vi "Material-ConfigPage-Launch.vi"(0 "Configuration Page VI Filepath":path, 5 "Config Dialog Messenger":refnum<class "FTW-Messenger-Actor.lvclass">, 11 "error in":errorcluster) -> (4 "PageID":string, 6 "Initialized?":bool, 8 "Page Messenger":refnum<class "FTW-Messenger-Actor.lvclass">, 15 "error out":errorcluster)   [LabVIEW 2013, in "Material-ConfigPage.lvclass"]
uses:
  Material-ConfigPage.lvclass
  Reuse Library/featherweight/Core/Messaging/Messenger.Actor/FTW-Messenger-Actor.lvclass
  Material-ConfigPage.lvclass/Material-ConfigPage.ctl
  Reuse Library/featherweight/Core/Messaging/Messenger/FTW-Messenger.lvclass
panel:
  # "Inputs"
  # "Outputs"
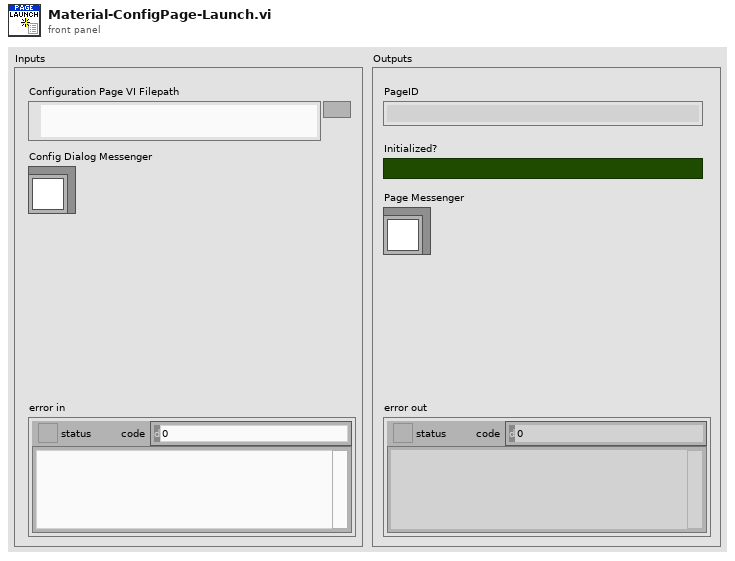
[diagram p1: front panel]
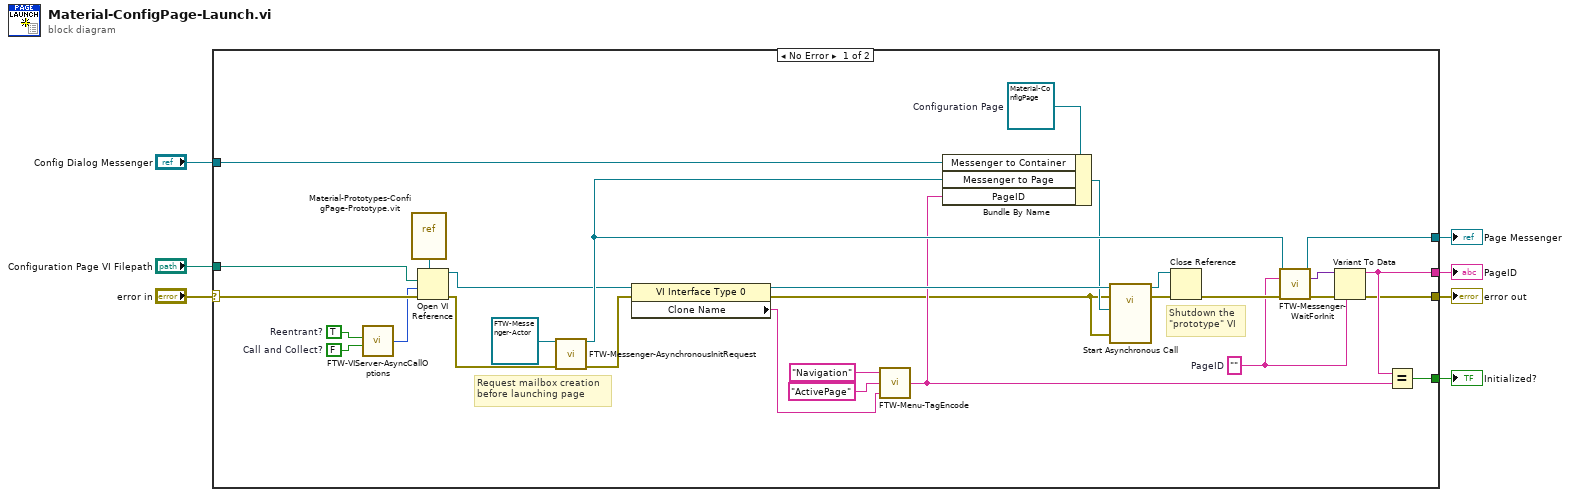
[diagram p0: block diagram]
diagram:
  n1 = case shown="No Error" "error in" {
    selector: "error in" -> [w36 w38]
    tunnel: [w10 w38] -> w7
    tunnel: "Configuration Page VI Filepath" -> [w37 _]
    tunnel: "Config Dialog Messenger" -> [w32 _]
    tunnel: [w25 _] -> w3
    tunnel: [w11 _] -> w2
    tunnel: [w24 _] -> w1
    frame No Error {
      w12 = ""  # PageID
      w28 = refnum<class "Material-ConfigPage.lvclass"> refnum  # Configuration Page
      w30 = FALSE  # Call and Collect?
      w31 = TRUE  # Reentrant?
      # "Shutdown the\n\"prototype\" VI"
      # "Request mailbox creation\nbefore launching page"
      n2 = call "FTW-VIServer-AsyncCallOptions.vi"("Call and Collect?"=w30, "Reentrant?"=w31) -> ("Open VI Ref Options"=w29:i32)  [unwired: 4 in]
      n3 = vi-ref "Material-Prototypes-ConfigPage-Prototype.vit"() -> (w35:refnum<vi>)
      n4 = Open VI Reference(type specifier VI Refnum (for type only)=w35, vi path=w37, options=w29, error in (no error)=w36) -> (vi reference=w21:refnum<vi>, error out=w20:errorcluster)  [unwired: 2 in]
      n5 = call-dynamic "FTW-Messenger-AsynchronousInitRequest.vi"("Messenger Type"=refnum<class "FTW-Messenger-Actor.lvclass"> refnum ("Interprocess Messenger"), "error in"=w20) -> ("Messenger"=w26:refnum<class "FTW-Messenger-Actor.lvclass">, "error out"=w22:errorcluster)  [unwired: 12 in]
      n6 = property class="VI Interface Type 0"(reference=w21, error in=w22) -> (reference out=w23:refnum<vi>, error out=w8:errorcluster, "Clone Name"=w17:string)
      n7 = call "FTW-Menu-TagEncode.vi"("Payload"=w17, "Command"="ActivePage", "Class"="Navigation") -> ("Tag"=w16:string)  [unwired: 1 in]
      n8 = Bundle By Name(cluster=w28, "Messenger to Container"=w32, "Messenger to Page"=w26, "PageID"=w16) -> (w9:refnum<class "Material-ConfigPage.lvclass">)
      n9 = call-by-ref "Start Asynchronous Call"(reference=w23, error in=w8, "Configuration Page"=w9, "error in"=w8) -> (reference out=w33:refnum<vi>, error out=w34:errorcluster)  [unwired: 13 in, 1 out]
      n10 = Close Reference(reference=w33, error in (no error)=w34) -> (error out=w27:errorcluster)
      n11 = call "FTW-Messenger-WaitForInit.vi"("Messenger"=w26, "Expected Response"=w12, "error in"=w27) -> ("Initialized Messenger"=w25:refnum<class "FTW-Messenger-Actor.lvclass">, "Response"=w13:variant, "error out"=w14:errorcluster)  [unwired: 9 in, 1 out]
      n12 = Variant To Data(error in=w14, type=w12, Variant=w13) -> (data=w11:string, error out=w10:errorcluster)
      n13 = Equal?(x=w11, y=w16) -> (x = y?=w24:bool)
    }
    frame Error {
    }
  }
  "error out" <- w7
  "Page Messenger" <- w3
  "PageID" <- w2
  "Initialized?" <- w1
